vi "Delete Key.vi"(8 "error in (no error)":errorcluster, 11 "CngKey in":refnum<k24>) -> (0 "error out":errorcluster, 3 "CngKey out":refnum<k24>)   [LabVIEW 2021, in "dotNET Crypto Key Management.lvlib"]
uses:
  dotNET Crypto Key Management.lvlib
  System.Core
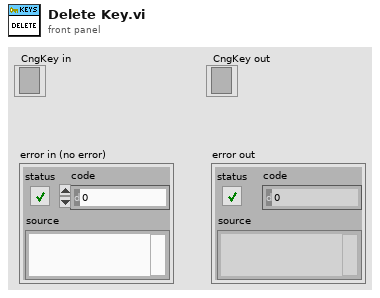
[diagram p1: front panel]
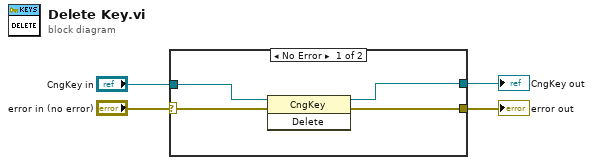
[diagram p0: block diagram]
diagram:
  n1 = case shown="No Error" "error in (no error)" {
    selector: "error in (no error)" -> [w5 w10]
    tunnel: [w8 w9] -> w4
    tunnel: "CngKey in" -> [w7 w9]
    tunnel: [w6 w10] -> w2
    frame No Error {
      n2 = invoke class="CngKey" method="Delete"(reference=w7, error in=w5) -> (reference out=w8:refnum<k24>, error out=w6:errorcluster)  [unwired: 1 in, 1 out]
    }
    frame Error {
    }
  }
  "CngKey out" <- w4
  "error out" <- w2
